vi "LABVIEW_Clase20190706_1.vi"() -> ()   [LabVIEW 2019]
uses:
  <vilib>/Instr/_visa.llb/VISA Configure Serial Port (Instr).vi
panel:
  out "Table":string[][](table)
  out "Waveform Chart":i32(graph)
  out "Meter":i32(knob) scale=0.0..255.0
  in  "stop":bool
  out "read buffer":string
  in  "parity (0:none)":enum16{"None", "Odd", "Even", "Mark", "Space"}(ring)
  in  "data bits (8)":u16=8 min=5 max=8 step=1
  in  "baud rate (9600)":u32=9600
  in  "VISA resource name":refnum<visa-resource-name>
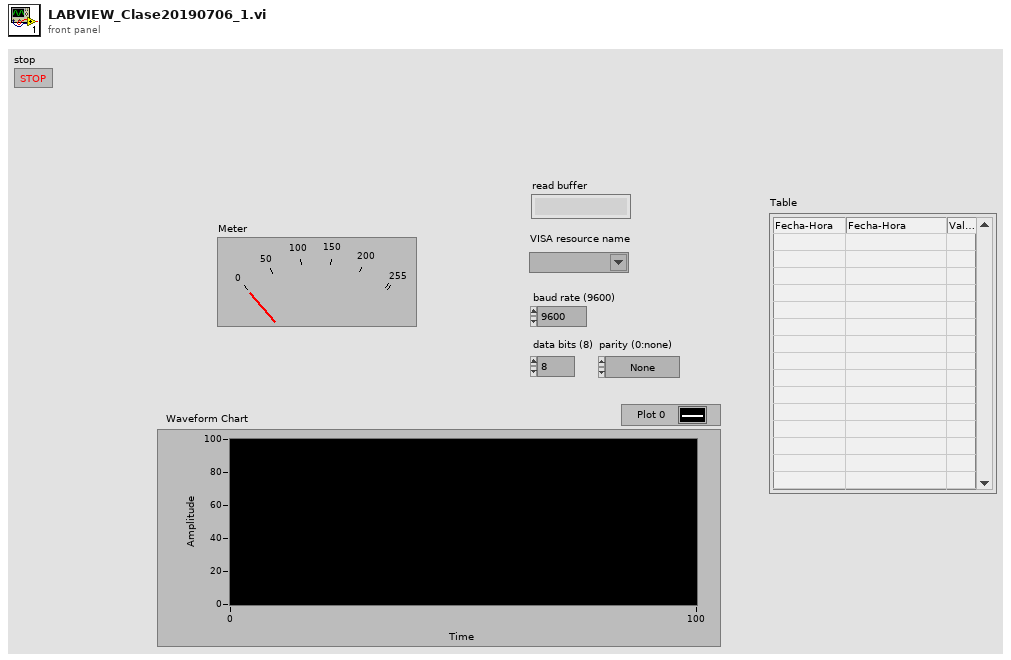
[diagram p1: front panel]
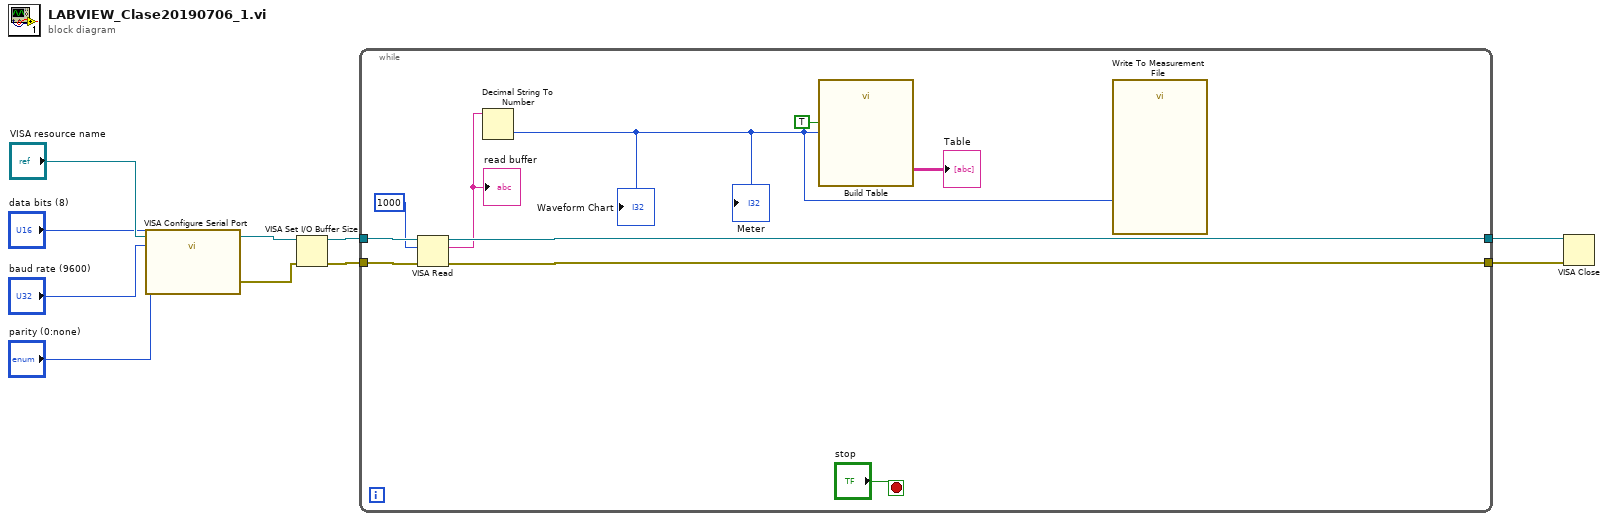
[diagram p0: block diagram]
diagram:
  n1 = call-poly "VISA Configure Serial Port"("VISA resource name"="VISA resource name", "baud rate (9600)"="baud rate (9600)", "data bits (8)"="data bits (8)", "parity (0:none)"="parity (0:none)") -> ("VISA resource name out"=w6:refnum<visa-resource-name>, "error out"=w5:errorcluster)  [unwired: 10 in]
  n2 = VISA Set I/O Buffer Size(VISA resource name=w6, error in (no error)=w5) -> (VISA resource name out=w3:refnum<visa-resource-name>, error out=w4:errorcluster)  [unwired: 2 in]
  n3 = while {
    tunnel: w4 -> [w20]
    tunnel: w3 -> [w19]
    tunnel: [w18] -> w2
    tunnel: [w17] -> w1
    stop <- "stop" stop-if-true
    n4 = VISA Read(VISA resource name=w19, byte count=u32 1000, error in (no error)=w20) -> (VISA resource name out=w18:refnum<visa-resource-name>, read buffer=w15:string, error out=w17:errorcluster)  [unwired: 1 out]
    "read buffer" <- w15
    n5 = Decimal String To Number(string=w15) -> (number=w12:i32)  [unwired: 2 in, 1 out]
    "Waveform Chart" <- w12
    "Meter" <- w12
    n6 = call "Build Table"("Include time data"=TRUE, "Signals"=w12) -> ("Table"=→"Table":string[][])  [unwired: 3 in, 6 out]
    n7 = call "Write To Measurement File"("Signals"=w12) -> ()  [unwired: 16 in, 3 out]
  }
  n8 = VISA Close(VISA resource name=w2, error in (no error)=w1) -> ()  [unwired: 1 out]
